vi "DMA.Scatter-Gather.Commit Blocks.vi"(8 "error in (no error)":errorcluster, 10 "Block Descriptors":T1[](array[typedef]) {"next descriptor ptr" format="%08x"; "data size" format="%08x"; "data ptr (upper)" format="%08x"; "data ptr (lower)" format="%08x"; "descriptor ptr (aligned)" format="%08x"; "descriptor size" format="%08x"; "descriptor ptr (VISA)" format="%08x"}, 11 "GE 5565PIORC in":refnum<class "GE 5565PIORC Old.lvclass">) -> (0 "error out":errorcluster, 2 "Block Descriptors out":T1[](array[typedef]) {"next descriptor ptr" format="%08x"; "data size" format="%08x"; "data ptr (upper)" format="%08x"; "data ptr (lower)" format="%08x"; "descriptor ptr (aligned)" format="%08x"; "descriptor size" format="%08x"; "descriptor ptr (VISA)" format="%08x"}, 3 "GE 5565PIORC out":refnum<class "GE 5565PIORC Old.lvclass">)   [LabVIEW 2016, in "GE 5565PIORC Old.lvclass"]
uses:
  GE 5565PIORC Old.lvclass
  Controls/DMA Block Descriptor.ctl
  GE 5565PIORC Old.lvclass/GE 5565PIORC Old.ctl
  <vilib>/Instr/_visa.llb/VISA Register Access Address Space.ctl
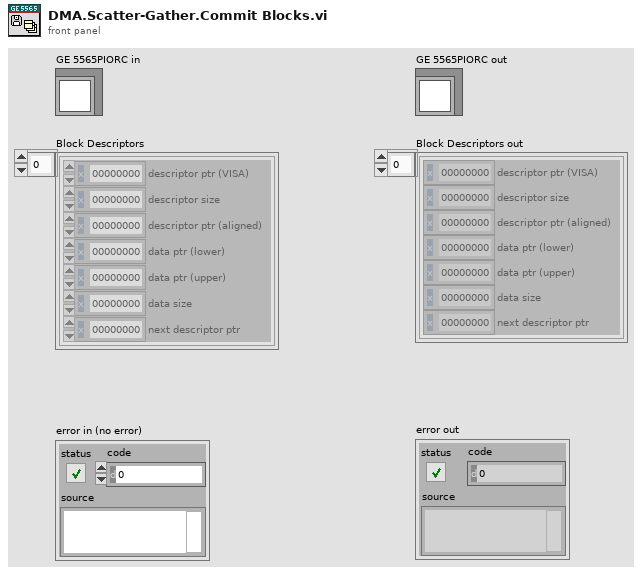
[diagram p1: front panel]
types:
  T1 = typedef "GE 5565PIORC Old.lvclass/DMA Block Descriptor.ctl" = cluster{"descriptor ptr (VISA)":u32, "descriptor size":u32, "descriptor ptr (aligned)":u32, "data ptr (lower)":u32, "data ptr (upper)":u32, "data size":u32, "next descriptor ptr":u32}
  T2 = typedef "VISA Register Access Address Space.ctl" = u16
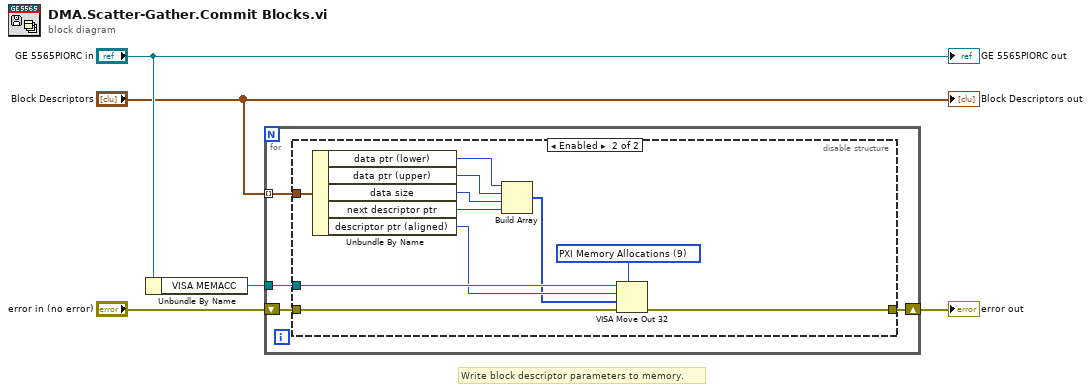
[diagram p0: block diagram]
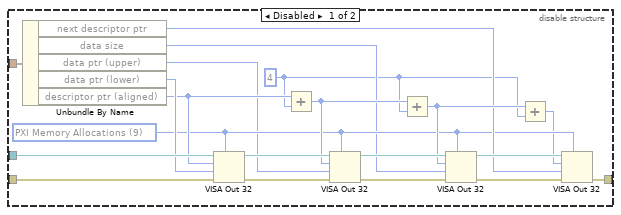
[diagram p2: hidden frame]
diagram:
  # "Write block descriptor parameters to memory."
  n1 = Unbundle By Name("GE 5565PIORC in") -> ("VISA MEMACC"=w4:refnum<visa-resource-name>)
  n2 = for {
    tunnel: "Block Descriptors" -> [w9] mode=indexing
    tunnel: w4 -> [w7]
    shift-right: [w6] -> w1
    shift-left: "error in (no error)" -> [w8]
    n3 = disable-structure shown="Enabled" {
      disable-tunnel: w9 -> [w29 w40]
      disable-tunnel: w8 -> [w28 w39]
      disable-tunnel: w7 -> [w27 w38]
      disable-tunnel: [w18 w35] -> w6
      frame Disabled {
        w14 = T2 9 items=["VXI/VME A16"=1, "VXI/VME A24"=2, "VXI/VME A32"=3, "VXI/VME A64"=4, "PXI Memory Allocations"=9, "PXI Configuration"=10, "PXI BAR0"=11, "PXI BAR1"=12, "PXI BAR2"=13, "PXI BAR3"=14, "PXI BAR4"=15, "PXI BAR5"=16] ("Address Space")
        w10 = u32 4 ("y")
        n4 = Unbundle By Name(w29) -> ("next descriptor ptr"=w15:u32, "data size"=w12:u32, "data ptr (upper)"=w13:u32, "data ptr (lower)"=w26:u32, "descriptor ptr (aligned)"=w25:u32)
        n5 = VISA Out 32(7:w14, 8:w28, 9:w26, 10:w25, 11:w27) -> (0:w21:errorcluster, 3:w24:refnum<visa-resource-name>)
        n6 = Add(x=w25, y=w10) -> (x+y=w17:u32)
        n7 = VISA Out 32(7:w14, 8:w21, 9:w13, 10:w17, 11:w24) -> (0:w20:errorcluster, 3:w23:refnum<visa-resource-name>)
        n8 = Add(x=w17, y=w10) -> (x+y=w16:u32)
        n9 = VISA Out 32(7:w14, 8:w20, 9:w12, 10:w16, 11:w23) -> (0:w19:errorcluster, 3:w22:refnum<visa-resource-name>)
        n10 = Add(x=w16, y=w10) -> (x+y=w11:u32)
        n11 = VISA Out 32(7:w14, 8:w19, 9:w15, 10:w11, 11:w22) -> (0:w18:errorcluster)  [unwired: 1 out]
      }
      frame Enabled {
        w36 = T2 9 items=["VXI/VME A16"=1, "VXI/VME A24"=2, "VXI/VME A32"=3, "VXI/VME A64"=4, "PXI Memory Allocations"=9, "PXI Configuration"=10, "PXI BAR0"=11, "PXI BAR1"=12, "PXI BAR2"=13, "PXI BAR3"=14, "PXI BAR4"=15, "PXI BAR5"=16] ("Address Space")
        n12 = Unbundle By Name(w40) -> ("data ptr (lower)"=w30:u32, "data ptr (upper)"=w31:u32, "data size"=w32:u32, "next descriptor ptr"=w33:u32, "descriptor ptr (aligned)"=w37:u32)
        n13 = Build Array(w30, w31, w32, w33) -> (w34:u32[])
        n14 = VISA Move Out 32(7:w36, 8:w39, 9:w34, 10:w37, 11:w38) -> (0:w35:errorcluster)  [unwired: 1 out]
      }
    }
  }
  "error out" <- w1
  "GE 5565PIORC out" <- "GE 5565PIORC in"
  "Block Descriptors out" <- "Block Descriptors"
